vi "exportLvDllNoDynamic.vi"(11 "ArrayIn":dbl[](array[numeric])) -> (3 "ArrayOut":dbl[](array[numeric]))   [LabVIEW 2020]
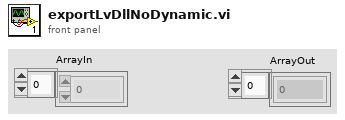
[diagram p1: front panel]
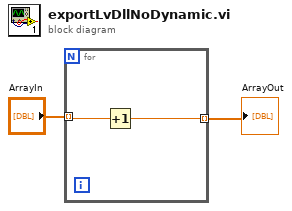
[diagram p0: block diagram]
diagram:
  n1 = for {
    tunnel: "ArrayIn" -> [w4] mode=indexing
    tunnel: [w3] -> w1 mode=indexing
    n2 = Increment(x=w4) -> (x+1=w3:dbl)
  }
  "ArrayOut" <- w1
